vi "Fetch Value.vi"(7 "PV name":string, 8 "error in":errorcluster, 11 "Server in":refnum<class "Server.lvclass">) -> (0 "error out":errorcluster, 2 "Value out":refnum<class "Value.lvclass">, 3 "Server out":refnum<class "Server.lvclass">)   [LabVIEW 2020, in "Server.lvlib" / "Server.lvclass"]
uses:
  Server.lvclass
  Value/Value/Value.lvclass
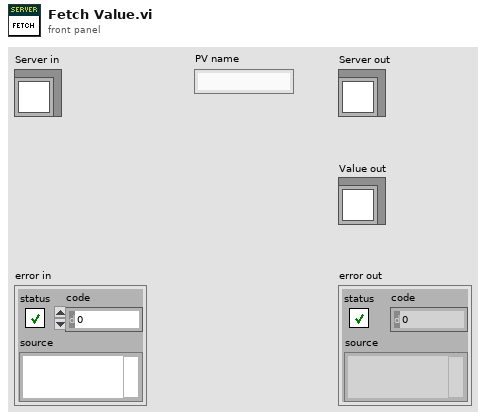
[diagram p1: front panel]
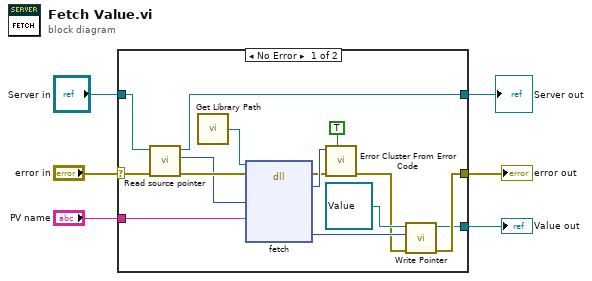
[diagram p0: block diagram]
diagram:
  n1 = case shown="No Error" "error in" {
    selector: "error in" -> [w21 w23]
    tunnel: [w8 w23] -> w4
    tunnel: [w16 w22] -> w5
    tunnel: "Server in" -> [w20 w22]
    tunnel: "PV name" -> [w15 _]
    tunnel: [w7 _] -> w1
    frame No Error {
      n2 = call "Read source pointer.vi"("error in (no error)"=w21, "Server in"=w20) -> ("error out"=w19:errorcluster, "source pointer"=w17:i64, "Server out"=w16:refnum<class "Server.lvclass">)  [unwired: 7 in]
      n3 = call "Get Library Path.vi"() -> ("Path"=w18:path)  [unwired: 1 in]
      n4 = dll-call lib="?" fn="fetch"(path in=w18, error in=w19, "source"=w17, "pv_name"=w15) -> (error out=w12:errorcluster, "ret_code"=w13:i32, "value"=w10:i64)  [unwired: 4 in, 1 out]
      n5 = call <vilib>:"Error Cluster From Error Code.vi"("show call chain? (False)"=TRUE, "error in (no error)"=w12, "error code (0)"=w13) -> ("error out"=w9:errorcluster)  [unwired: 6 in]
      n6 = call-dynamic "Write Pointer.vi"("error in (no error)"=w9, "Pointer"=w10, "Value in"=refnum<class "Value.lvclass"> refnum) -> ("error out"=w8:errorcluster, "Value out"=w7:refnum<class "Value.lvclass">)  [unwired: 7 in]
    }
    frame Error {
    }
  }
  "error out" <- w4
  "Server out" <- w5
  "Value out" <- w1
